vi "PS Control Launcher.vi"() -> ()   [LabVIEW 2025]
doc: "Author: Scott Hannahs <sth@magnet.fsu.edu>\n\nThis software is licensed for use under the “MIT License\"\nCopyright (c) 2025 Scott Hannahs, sth@sth@magnet.sthnet.net\n\nPermission is hereby granted, free of charge, to any person obtaining a copy of this software and associated documentation files (the \"Software\"), to deal in the Software without restriction, including without limitation the rights to use, copy, modify, merge, publish, distribute, sublicense, and/or sell copies of the Software, and to permit persons to whom the Software is furnished to do so, subject to the following conditions: The above copyright notice and this permission notice shall be included in all copies or substantial portions of the Software.\n\nTHE SOFTWARE IS PROVIDED \"AS IS\", WITHOUT WARRANTY OF ANY KIND, EXPRESS OR IMPLIED, INCLUDING BUT NOT LIMITED TO THE WARRANTIES OF MERCHANTABILITY, FITNESS FOR A PARTICULAR PURPOSE AND NONINFRINGEMENT. IN NO EVENT SHALL THE AUTHORS OR COPYRIGHT HOLDERS BE LIABLE FOR ANY CLAIM, DAMAGES OR OTHER LIABILITY, WHETHER IN AN ACTION OF CONTRACT, TORT OR OTHERWISE, ARISING FROM, OUT OF OR IN CONNECTION WITH THE SOFTWARE OR THE USE OR OTHER DEALINGS IN THE SOFTWARE."
uses:
  PS Driver/AMI 4xx/PS Driver AMI4xx.lvclass
  PS Control Actor.lvclass
  PS Control Persistence Actor/PS Control Persistence Actor.lvclass
  <userlib>/_OpenG.lib/appcontrol/appcontrol.llb/openg_application_control.lvlib
panel:
  in  "stop":bool
  out "error out":errorcluster
  # "Starting PS Control"
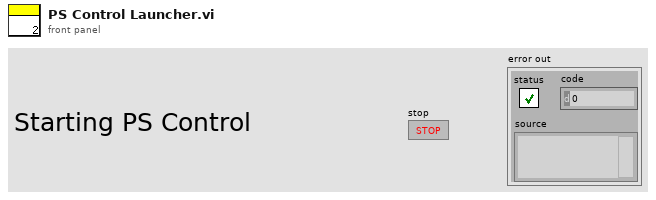
[diagram p1: front panel]
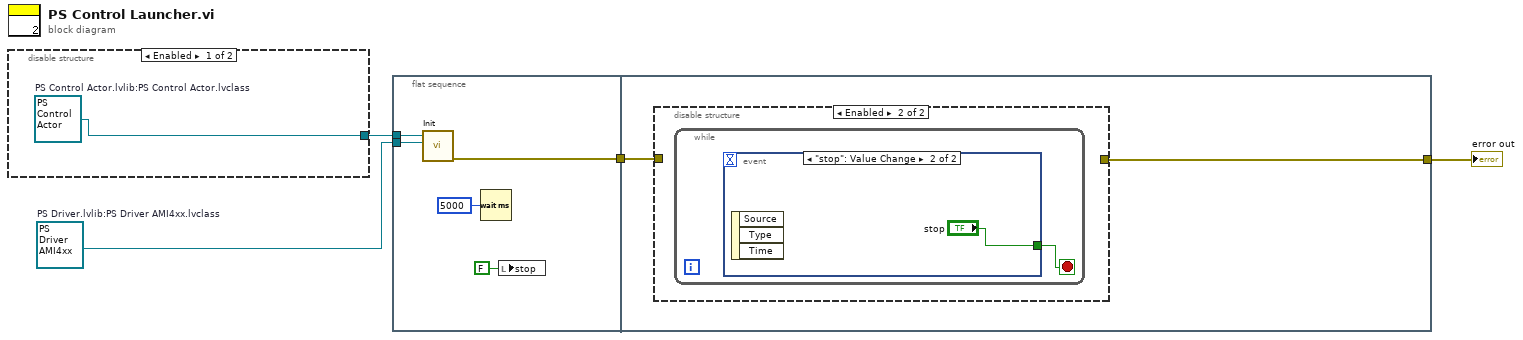
[diagram p0: block diagram]
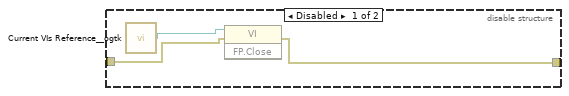
[diagram p2: hidden frame]
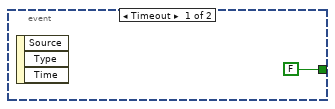
[diagram p3: hidden frame]
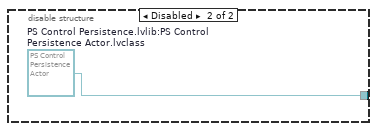
[diagram p4: hidden frame]
diagram:
  w3 = refnum<class "PS Driver AMI4xx.lvclass"> refnum  # PS Driver.lvlib:PS Driver AMI4xx.lvclass
  n1 = disable-structure shown="Enabled" {
    disable-tunnel: [w5 w6] -> w4
    frame Enabled {
      w5 = refnum<class "PS Control Actor.lvclass"> refnum  # PS Control Actor.lvlib:PS Control Actor.lvclass
    }
    frame Disabled {
      w6 = refnum<class "PS Control Persistence Actor.lvclass"> refnum  # PS Control Persistence.lvlib:PS Control Persistence Actor.lvclass
    }
  }
  n2 = flat-sequence {
    tunnel: w4 -> [w11]
    tunnel: w3 -> [w10]
    tunnel: [w8] -> w2
    tunnel: w2 -> [w13]
    tunnel: [w12] -> w1
    frame #0 {
      n3 = call "Init.vi"("PS Driver.lvlib:PS Driver.lvclass"=w10, "PS Control Actor in"=w11) -> ("error out"=w8:errorcluster)  [unwired: 8 in, 1 out]
      n4 = Wait (ms)(milliseconds to wait=u32 5000) -> ()  [unwired: 1 out]
      n5 = local write "stop"(FALSE ("stop")) -> ()
    }
    frame #1 {
      n6 = disable-structure shown="Enabled" {
        disable-tunnel: w13 -> [w15 _]
        disable-tunnel: [w14 _] -> w12
        frame Disabled {
          n7 = call <userlib>:"Current VIs Reference__ogtk.vi"() -> ("Current VI's reference"=w16:refnum<vi>)  [unwired: 5 in]
          n8 = invoke class="VI" method="FP.Close"(reference=w16, error in=w15) -> (error out=w14:errorcluster)  [unwired: 1 in, 2 out]
        }
        frame Enabled {
          n9 = while {
            stop <- w17 stop-if-true
            n10 = event shown="[1] \"stop\": Value Change" {
              selector: _ -> [_ _]
              dyn-events: _ -> [_ _]
              timeout: _ -> [_ _]
              tunnel: [FALSE "stop"] -> w17
              event Timeout {
                n11 = event-data() -> ()  [unwired: 1 in, 3 out]
              }
              event "stop": Value Change {
                n12 = event-data() -> ()  [unwired: 1 in, 3 out]
              }
            }
          }
        }
      }
    }
  }
  "error out" <- w1
